vi "Unflatten XML to Variant (PVI).vi"(8 "error in (no error)":errorcluster, 10 "XML":string, 11 "Variant in (for type and default data)":variant) -> (0 "error out":errorcluster, 3 "Variant out":variant)   [LabVIEW 2018, in "XML Config.lvlib"]
doc: "This VI is used to facilitate saving XML files of arbitrary simple clusters (i.e one\nthat does not contain arrays of clusters) as config files and then reading them\nback even though the cluster may have been updated (may added or removed\ncontrols from the cluster).Unflattens \"XML\" into the type of data given by \"Variant in\".\nValues in \"Variant in\" that have matching names with the \"XML\" will\nbe replaced by values from the XML.\n\nThe \"XML\" must be generated using the Flatten to XML (PVI).vi. If a control\nin the \"Variant in\" does not exist in the \"XML\", then the \"Variant in\" value for\nthat control will be retained and output to the \"Variant out\"."
uses:
  XML Config.lvlib
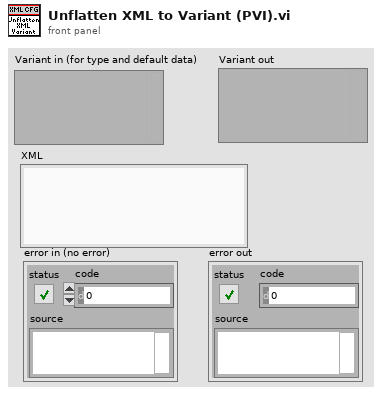
[diagram p1: front panel]
types:
  T1 = cluster{"Name Paths":cluster{"Name Path":string[]}[], "Values":string[]}
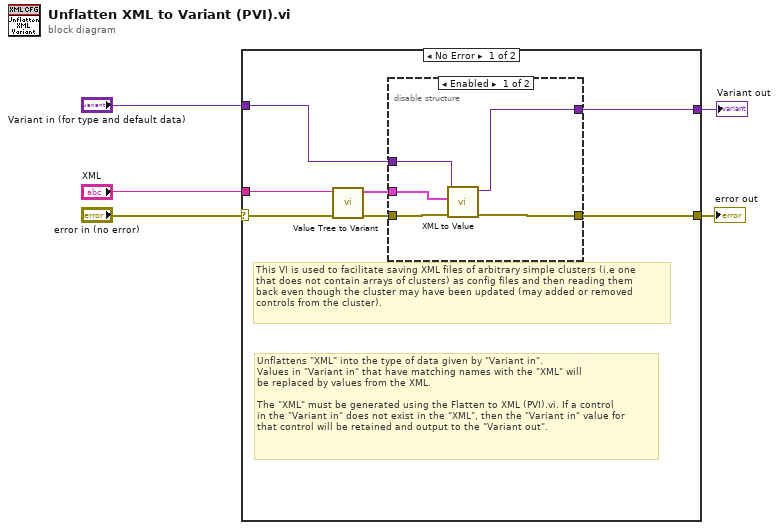
[diagram p0: block diagram]
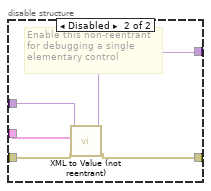
[diagram p2: hidden frame]
diagram:
  n1 = case shown="No Error" "error in (no error)" {
    selector: "error in (no error)" -> [w7 w24]
    tunnel: [w11 w24] -> w5
    tunnel: "XML" -> [w10 _]
    tunnel: [w8 w23] -> w3
    tunnel: "Variant in (for type and default data)" -> [w6 w23]
    frame No Error {
      # "This VI is used to facilitate saving XML files of arbitrary simple clusters (i.e one\nthat does not contain arrays of clusters) as config files and then reading them\nback even though the cluster may have been updated (may added or removed\ncontrols from the cluster)."
      # "Unflattens \"XML\" into the type of data given by \"Variant in\".\nValues in \"Variant in\" that have matching names with the \"XML\" will\nbe replaced by values from the XML.\n\nThe \"XML\" must be generated using the Flatten to XML (PVI).vi. If a control\nin the \"Variant in\" does not exist in the \"XML\", then the \"Variant in\" value for\nthat control will be retained and output to the \"Variant out\"."
      n2 = call "Value Tree to Variant.vi"("error in (no error)"=w7, "XML in"=w10) -> ("error out"=w12:errorcluster, "Value Tree"=w9:T1)  [unwired: 8 in]
      n3 = disable-structure shown="Enabled" {
        disable-tunnel: w12 -> [w17 w19]
        disable-tunnel: [w16 w20] -> w11
        disable-tunnel: w9 -> [w15 w18]
        disable-tunnel: [w14 w21] -> w8
        disable-tunnel: w6 -> [w13 w22]
        frame Enabled {
          n4 = call "XML to Value.vi"("error in (no error)"=w17, "Value Tree"=w15, "Variant in"=w13) -> ("error out"=w16:errorcluster, "Variant out"=w14:variant)  [unwired: 7 in]
        }
        frame Disabled {
          # "Enable this non-reentrant\nfor debugging a single\nelementary control"
          n5 = call "XML to Value (not reentrant).vi"("error in (no error)"=w19, "Value Tree"=w18, "Variant in"=w22) -> ("error out"=w20:errorcluster, "Variant out"=w21:variant)  [unwired: 7 in]
        }
      }
    }
    frame Error {
    }
  }
  "error out" <- w5
  "Variant out" <- w3
